vi "Update.vi"(9 "Column":i32, 10 "Row":i32, 11 "64 in":refnum<class "Border.lvclass">) -> (3 "64 out":refnum<class "Border.lvclass">)   [LabVIEW 2015, in "Border.lvclass"]
uses:
  Border.lvclass
  Border Type.ctl
  Common/Position.ctl
  Border.lvclass/Border.ctl
  SubVIs/Read-Only Globals.vi
  SubVIs/Globals (private).vi
  Square/Square.lvclass
  Common/Common.lvlib
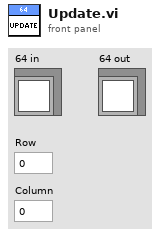
[diagram p1: front panel]
types:
  T1 = typedef "Common.lvlib/Position.ctl" = cluster{"Column":i32, "Row":i32}
  T2 = typedef "Border.lvclass/Border Type.ctl" = enum16{"Starter", "Assassin", "Line Starter", "ELine", "WLine", "StartPatrol", "Patrol", "Wall"}
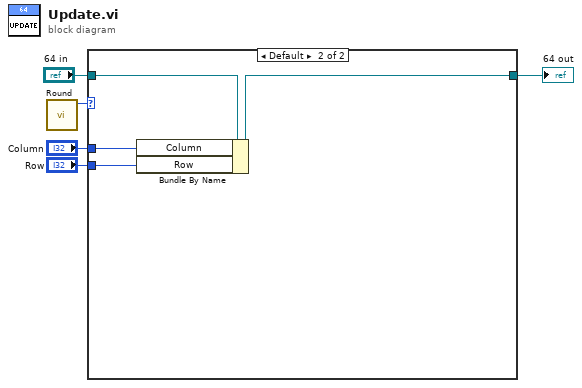
[diagram p0: block diagram]
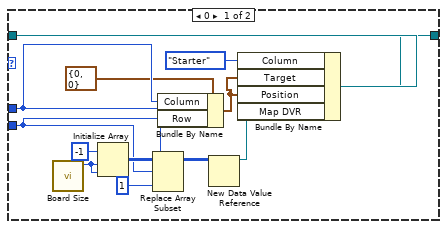
[diagram p2: hidden frame]
diagram:
  n1 = call "Round.vi"() -> ("Round"=w3:i32)  [unwired: 11 in]
  n2 = case shown="Default" w3 {
    tunnel: "64 in" -> [w18 w22]
    tunnel: [w17 w21] -> w4
    tunnel: "Row" -> [w8 w19]
    tunnel: "Column" -> [w9 w20]
    frame 0 {
      n3 = call "Board Size.vi"() -> ("Board Size"=w14:i32)  [unwired: 11 in]
      n4 = Initialize Array(-1, w14, w14) -> (w13:i32[][])
      n5 = Replace Array Subset(array=w13, new element=1 ("new element/subarray"), index (row)=w8, index (col)=w9) -> (w11:i32[][])
      n6 = Bundle By Name(cluster=T1 {"Column"=0, "Row"=0} ("Center"), "Column"=w9, "Row"=w8) -> (w6:T1)
      n7 = New Data Value Reference(data value=w11) -> (data value reference=w12:refnum<data-value>)  [unwired: 1 in, 1 out]
      n8 = Bundle By Name(cluster=w18, "Column"=Border_Type."Starter" ("Type"), "Target"=w6, "Position"=w6, "Map DVR"=w12) -> (w17:refnum<class "Border.lvclass">)
    }
    frame Default {
      n9 = Bundle By Name(cluster=w22, "Column"=w20, "Row"=w19) -> (w21:refnum<class "Border.lvclass">)
    }
  }
  "64 out" <- w4
